vi "显示字符串的ASCII值（空格分隔）.vi"(11 "接收字符串（正常显示）":string) -> (3 "显示字符串（正常显示HEX)":string)   [LabVIEW 2012]
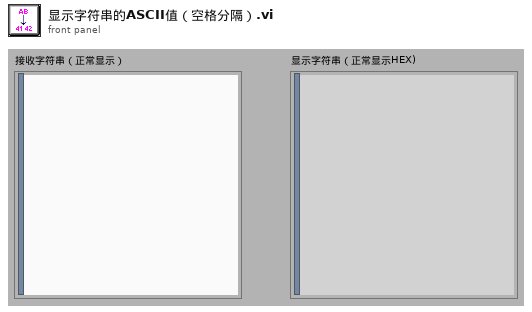
[diagram p1: front panel]
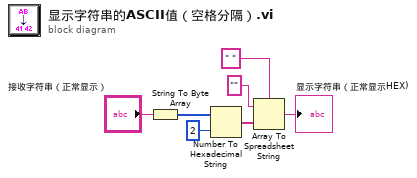
[diagram p0: block diagram]
diagram:
  n1 = String To Byte Array(string="接收字符串（正常显示）") -> (unsigned byte array=w6:u8[])
  n2 = Number To Hexadecimal String(1:i16 2 ("宽度(-)"), 2:w6) -> (0:w4:string[])
  n3 = Array To Spreadsheet String(delimiter (Tab)=" " ("分隔符(Tab)"), array=w4, 3:"" ("格式字符串")) -> (spreadsheet string=→"显示字符串（正常显示HEX)":string)
